vi "PH_Switch_USB.set i Attr.vi"(0 "i ref in":refnum<vi>, 5 "error in (no error)":errorcluster) -> (14 "i ref out":refnum<vi>, 17 "i Attributes":T1={"GUI Refs"={"GUI-Knob"=refnum, "Delete"=refnum}, "Switch"={"GUI Ref"=refnum, "Service name"="N/A", "Array No."=9999, "caption"="", "Status"=0}, "True-Sensor"={"GUI Ref"=refnum, "Service name"="N/A", "Array No."=9999, "caption"="", "Status"=0}, "False-Sensor"={"GUI Ref"=refnum, "Service name"="N/A", "Array No."=9999, "caption"="", "Status"=0}} {"False-Sensor"."Status" items=["no info", "off/false/out", "on/true/in", "Failure", "Alarm", "Status 1", "Status 2", "Status 3"]; "True-Sensor"."Status" items=["no info", "off/false/out", "on/true/in", "Failure", "Alarm", "Status 1", "Status 2", "Status 3"]; "Switch"."Status" items=["no info", "off/false/out", "on/true/in", "Failure", "Alarm", "Status 1", "Status 2", "Status 3"]}, 19 "error out":errorcluster)   [LabVIEW 2014, in "PH_Switch_USB.lvlib"]
doc: "This VI reads the database and stores the inform,ation to own attributes."
uses:
  PH_Switch_USB.lvlib
  PH_Switch_USB.i attribute.ctl
  PH_Basics/PH_StatusHandler/PH_StatusHandler.Status.ctl
  PH_Basics/PH_StatusHandler/PH_StatusHandler.lvlib
  PH_Basics/PH_Common/PH_Common.lvlib
  CS_Core/CSSystem/CSSystemLib/CSSystemLib.lvlib
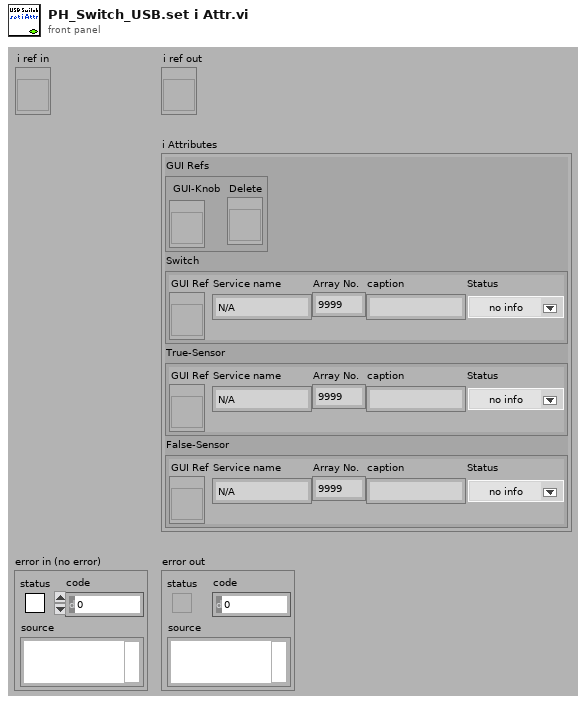
[diagram p1: front panel]
types:
  T1 = typedef "PH_Switch_USB.lvlib/PH_Switch_USB.i attribute.ctl" = cluster{"GUI Refs":cluster{"GUI-Knob":refnum<vi>, "Delete":refnum<vi>}, "Switch":cluster{"GUI Ref":refnum<vi>, "Service name":string, "Array No.":i16, "caption":string, "Status":T2}, "True-Sensor":cluster{"GUI Ref":refnum<vi>, "Service name":string, "Array No.":i16, "caption":string, "Status":T2}, "False-Sensor":cluster{"GUI Ref":refnum<vi>, "Service name":string, "Array No.":i16, "caption":string, "Status":T2}}
  T2 = typedef "PH_StatusHandler.lvlib/PH_StatusHandler.Status.ctl" = i16
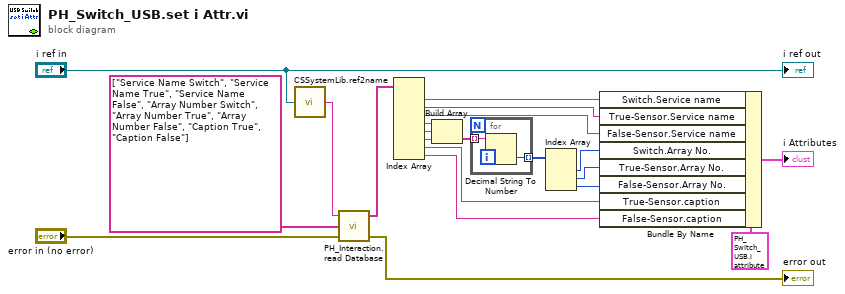
[diagram p0: block diagram]
diagram:
  n1 = call "CSSystemLib.ref2name.vi"("obj refnum"="i ref in") -> ("name"=w3:string)
  n2 = call "PH_Interaction.read Database.vi"("error in (no error)"="error in (no error)", "Strings to search for"=string[] ["Service Name Switch", "Service Name True", "Service Name False", "Array Number Switch", "Array Number True", "Array Number False", "Caption True", "Caption False"], "DB Entry to read"=w3) -> ("error out"=→"error out":errorcluster, "Values"=w13:string[])  [unwired: 1 in]
  n3 = Index Array(array=w13) -> (element #1=w6:string, element #2=w5:string, element #3=w4:string, element #4=w12:string, element #5=w11:string, element #6=w10:string, element #7=w9:string, element #8=w8:string)  [unwired: 8 in]
  n4 = Build Array(w12, w11, w10) -> (w7:string[])
  n5 = for {
    tunnel: [w23] -> w20 mode=indexing
    tunnel: w7 -> [w22] mode=indexing
    n6 = Decimal String To Number(string=w22) -> (number=w23:i32)  [unwired: 2 in, 1 out]
  }
  n7 = Index Array(array=w20) -> (element #1=w17:i32, element #2=w18:i32, element #3=w19:i32)  [unwired: 3 in]
  n8 = Bundle By Name(cluster=T1 {"GUI Refs"={"GUI-Knob"=refnum, "Delete"=refnum}, "Switch"={"GUI Ref"=refnum, "Service name"="", "Array No."=0, "caption"="", "Status"=0}, "True-Sensor"={"GUI Ref"=refnum, "Service name"="", "Array No."=0, "caption"="", "Status"=0}, "False-Sensor"={"GUI Ref"=refnum, "Service name"="", "Array No."=0, "caption"="", "Status"=0}} ("i attribute"), "Switch.Service name"=w6, "True-Sensor.Service name"=w5, "False-Sensor.Service name"=w4, "Switch.Array No."=w17, "True-Sensor.Array No."=w18, "False-Sensor.Array No."=w19, "True-Sensor.caption"=w9, "False-Sensor.caption"=w8) -> (→"i Attributes":T1)
  "i ref out" <- "i ref in"
